vi "ManipSetIntaking.vi"(2 "Reinit":bool, 3 "Parameter String":string) -> (0 "Error Out":errorcluster, 1 "Advance Trigger":bool)   [LabVIEW 2023]
doc: "This VI switches whether the robot intake is on or off in autonomous.\n\nParameters:\n1. \"on\" or \"off\""
uses:
  SafeParser_String.vi
  GlobalDriverStationCommands.vi
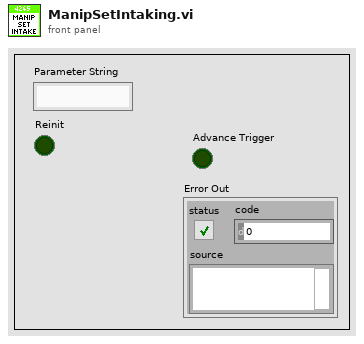
[diagram p1: front panel]
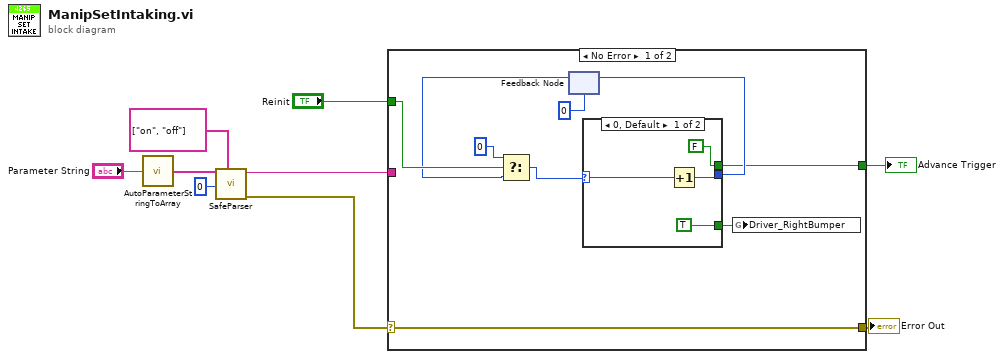
[diagram p0: block diagram]
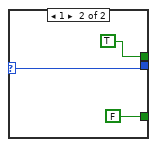
[diagram p2: hidden frame]
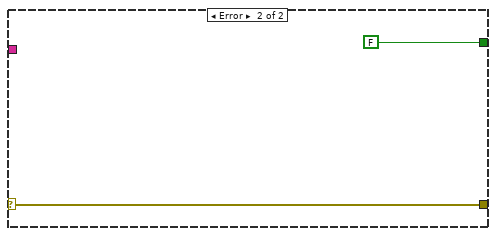
[diagram p3: hidden frame]
diagram:
  n1 = call "AutoParameterStringToArray.vi"("Parameter String"="Parameter String") -> ("Parsed Parameters"=w4:string[])
  n2 = call-poly "SafeParser.vi"("Allowed Values"=string[] ["on", "off"], "Array Index"=0 ("Parameter Index"), "String Array"=w4) -> ("Error Out"=w2:errorcluster, "Typecast Value"=w6:string)  [unwired: 7 in]
  n3 = case shown="No Error" w2 {
    selector: w2 -> [w18 w27]
    tunnel: [w10 FALSE] -> w9
    tunnel: [w18 w27] -> w8
    tunnel: w6 -> [_ _]
    tunnel: "Reinit" -> [w14 _]
    frame No Error {
      n4 = feedback #1(0) -> (w12:i32)
      n5 = Select(t=0, s=w14, f=w12) -> (s? t:f=w11:i32)
      n6 = case shown="0, Default" w11 {
        selector: w11 -> [w22 w25]
        tunnel: [w21 w25] -> w16
        tunnel: [TRUE FALSE] -> w15
        tunnel: [FALSE TRUE] -> w10
        frame 0, Default {
          n7 = Increment(x=w22) -> (x+1=w21:i32)
        }
        frame 1 {
        }
      }
      n8 = feedback-in #1(w16) -> ()
      n9 = global write "GlobalDriverStationCommands.vi" "Driver_RightBumper"(w15) -> ()
    }
    frame Error {
    }
  }
  "Advance Trigger" <- w9
  "Error Out" <- w8
